vi "Diamond Target Analysis.vi"(10 "gun tracking mode":T1, 11 "Diamond Targets":T4[](array[typedef])) -> (3 "Targetting Output":T3)   [LabVIEW 2011]
uses:
  Diamond Target Output.ctl
  Rectangle Position.ctl
  Target Confidence.ctl
  Camera State.ctl
  gun/gun_tracking_mode.ctl
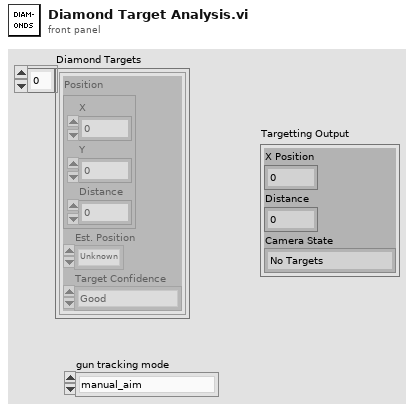
[diagram p1: front panel]
types:
  T1 = typedef "gun_tracking_mode.ctl" = enum16{"manual_aim", "auto_aim_camera", "preset_center_field", "preset_right_pocket", "preset_left_pocket", "align_center", "align_center_backwards", "auto_aim_key", "align_fold", "auton_custom", "preset_pass", "auto_aim_auton"}
  T2 = typedef "Camera State.ctl" = enum16{"No Targets", "Low Confidence", "Medium Confidence", "High Confidence", "Camera Error"}
  T3 = cluster{"X Position":dbl, "Distance":dbl, "Camera State":T2}
  T4 = typedef "Diamond Target Output.ctl" = cluster{"Position":cluster{"X":dbl, "Y":dbl, "Distance":dbl}, "Est. Position":T5, "Target Confidence":T6}
  T5 = typedef "Rectangle Position.ctl" = enum16{"Unknown", "Top", "Right", "Left", "Bottom"}
  T6 = typedef "Target Confidence.ctl" = enum16{"Good", "Good-Clipped Y", "Marginal-Clipped X"}
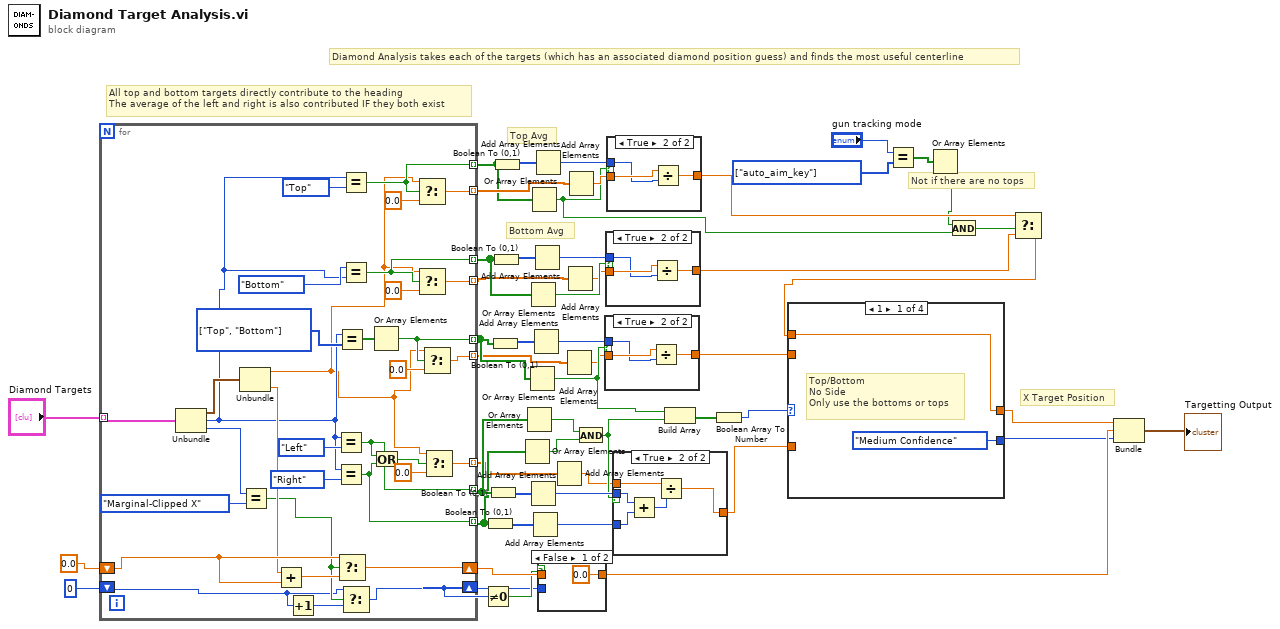
[diagram p0: block diagram]
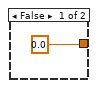
[diagram p2: hidden frame]
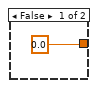
[diagram p3: hidden frame]
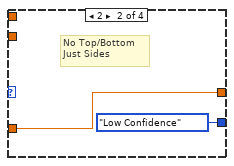
[diagram p4: hidden frame]
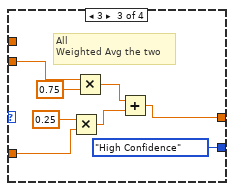
[diagram p5: hidden frame]
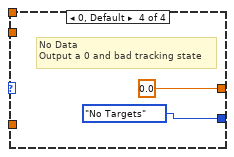
[diagram p6: hidden frame]
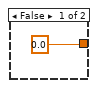
[diagram p7: hidden frame]
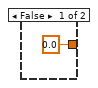
[diagram p8: hidden frame]
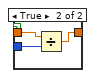
[diagram p9: hidden frame]
diagram:
  w8 = T1[] [enum."auto_aim_key"] items=["manual_aim", "auto_aim_camera", "preset_center_field", "preset_right_pocket", "preset_left_pocket", "align_center", "align_center_backwards", "auto_aim_key", "align_fold", "auton_custom", "preset_pass", "auto_aim_auton"]
  # "Diamond Analysis takes each of the targets (which has an associated diamond position guess) and finds the most useful centerline"
  # "Not if there are no tops"
  # "Top Avg"
  # "Bottom Avg"
  # "X Target Position"
  # "All top and bottom targets directly contribute to the heading\nThe average of the left and right is also contributed IF they both exist"
  n1 = for {
    tunnel: "Diamond Targets" -> [w85] mode=indexing
    tunnel: [w68] -> w37 mode=indexing
    tunnel: [w66] -> w39 mode=indexing
    shift-right: [w77] -> w48
    shift-left: 0.0 -> [w75]
    shift-right: [w73] -> w46
    shift-left: 0 -> [w70]
    tunnel: [w69] -> w38 mode=indexing
    tunnel: [w65] -> w25 mode=indexing
    tunnel: [w63] -> w23 mode=indexing
    tunnel: [w59] -> w15 mode=indexing
    tunnel: [w58] -> w16 mode=indexing
    tunnel: [w54] -> w11 mode=indexing
    tunnel: [w53] -> w10 mode=indexing
    w79 = T5[] [enum."Top", enum."Bottom"] items=["Unknown", "Top", "Right", "Left", "Bottom"]
    n2 = Unbundle(w85) -> ("Position"=w84:cluster{"X":dbl, "Y":dbl, "Distance":dbl}, "Est. Position"=w56:T5, "Target Confidence"=w83:T6)
    n3 = Unbundle(w84) -> ("X"=w52:dbl, "Distance"=w74:dbl)  [unwired: 1 out]
    n4 = Equal?(x=w83, y=Target_Confidence."Marginal-Clipped X") -> (x = y?=w72:bool)
    n5 = Add(x=w74, y=w75) -> (x+y=w76:dbl)
    n6 = Increment(x=w70) -> (x+1=w71:i32)
    n7 = Equal?(x=w56, y=Rectangle_Position."Left") -> (x = y?=w69:bool)
    n8 = Equal?(x=w56, y=Rectangle_Position."Right") -> (x = y?=w68:bool)
    n9 = Equal?(x=w56, y=w79) -> (x = y?=w78:bool[])
    n10 = Select(t=w75, s=w72, f=w76) -> (s? t:f=w77:dbl)
    n11 = Equal?(x=w56, y=Rectangle_Position."Top") -> (x = y?=w53:bool)
    n12 = Equal?(x=Rectangle_Position."Bottom" ("y"), y=w56) -> (x = y?=w58:bool)
    n13 = Select(t=w70, s=w72, f=w71) -> (s? t:f=w73:i32)
    n14 = Or Array Elements(Boolean array=w78) -> (logical OR=w66:bool)
    n15 = Or(x=w69, y=w68) -> (x .or. y?=w67:bool)
    n16 = Select(t=w52, s=w53, f=0.0) -> (s? t:f=w54:dbl)
    n17 = Select(t=w52, s=w58, f=0.0) -> (s? t:f=w59:dbl)
    n18 = Select(t=w52, s=w66, f=0.0) -> (s? t:f=w63:dbl)
    n19 = Select(t=w52, s=w67, f=0.0) -> (s? t:f=w65:dbl)
  }
  n20 = Not Equal To 0?(x=w46) -> (x != 0?=w47:bool)
  n21 = Boolean To (0,1)(Boolean=w37) -> (0, 1=w43:i16[])
  n22 = Boolean To (0,1)(Boolean=w38) -> (0, 1=w44:i16[])
  n23 = Boolean To (0,1)(Boolean=w39) -> (0, 1=w45:i16[])
  n24 = Boolean To (0,1)(Boolean=w16) -> (0, 1=w20:i16[])
  n25 = Boolean To (0,1)(Boolean=w10) -> (0, 1=w14:i16[])
  n26 = Or Array Elements(Boolean array=w37) -> (logical OR=w35:bool)
  n27 = Or Array Elements(Boolean array=w38) -> (logical OR=w36:bool)
  n28 = Or Array Elements(Boolean array=w39) -> (logical OR=w34:bool)
  n29 = Or Array Elements(Boolean array=w16) -> (logical OR=w18:bool)
  n30 = Add Array Elements(numeric array=w44) -> (sum=w41:i16)
  n31 = Or Array Elements(Boolean array=w10) -> (logical OR=w1:bool)
  n32 = Add Array Elements(numeric array=w43) -> (sum=w40:i16)
  n33 = Add Array Elements(numeric array=w45) -> (sum=w42:i16)
  n34 = Add Array Elements(numeric array=w20) -> (sum=w19:i16)
  n35 = Add Array Elements(numeric array=w14) -> (sum=w13:i16)
  n36 = case shown="False" w47 {
    tunnel: w48 -> [_ w89]
    tunnel: w46 -> [_ w88]
    tunnel: [0.0 w87] -> w27
    frame False {
    }
    frame True {
      n37 = Divide(x=w89, y=w88) -> (x/y=w87:dbl)
    }
  }
  n38 = Add Array Elements(numeric array=w25) -> (sum=w24:dbl)
  n39 = Add Array Elements(numeric array=w23) -> (sum=w22:dbl)
  n40 = Add Array Elements(numeric array=w15) -> (sum=w17:dbl)
  n41 = Add Array Elements(numeric array=w11) -> (sum=w12:dbl)
  n42 = And(x=w36, y=w35) -> (x .and. y?=w33:bool)
  n43 = case shown="True" w34 {
    tunnel: w22 -> [_ w93]
    tunnel: w42 -> [_ w92]
    tunnel: [0.0 w91] -> w30
    frame False {
    }
    frame True {
      n44 = Divide(x=w93, y=w92) -> (x/y=w91:dbl)
    }
  }
  n45 = case shown="True" w18 {
    tunnel: w17 -> [_ w97]
    tunnel: w19 -> [_ w96]
    tunnel: [0.0 w95] -> w5
    frame False {
    }
    frame True {
      n46 = Divide(x=w97, y=w96) -> (x/y=w95:dbl)
    }
  }
  n47 = case shown="True" w1 {
    tunnel: w12 -> [_ w101]
    tunnel: w13 -> [_ w100]
    tunnel: [0.0 w99] -> w6
    frame False {
    }
    frame True {
      n48 = Divide(x=w101, y=w100) -> (x/y=w99:dbl)
    }
  }
  n49 = case shown="True" w33 {
    tunnel: w41 -> [_ w107]
    tunnel: w40 -> [_ w106]
    tunnel: [0.0 w103] -> w29
    tunnel: w24 -> [_ w104]
    frame False {
    }
    frame True {
      n50 = Add(x=w107, y=w106) -> (x+y=w105:i16)
      n51 = Divide(x=w104, y=w105) -> (x/y=w103:dbl)
    }
  }
  n52 = Build Array(w34, w33) -> (w32:bool[])
  n53 = Boolean Array To Number(Boolean array=w32) -> (number=w31:u32)
  n54 = Equal?(x="gun tracking mode", y=w8) -> (x = y?=w7:bool[])
  n55 = Or Array Elements(Boolean array=w7) -> (logical OR=w2:bool)
  n56 = And(x=w2, y=w1) -> (x .and. y?=w3:bool)
  n57 = Select(t=w6, s=w3, f=w5) -> (s? t:f=w4:dbl)
  n58 = case shown="1" w31 {
    tunnel: [Camera_State."Medium Confidence" ("Camera State") Camera_State."Low Confidence" ("Camera State") Camera_State."High Confidence" ("Camera State") Camera_State."No Targets" ("Camera State")] -> w26
    tunnel: [w108 w110 w112 0.0] -> w28
    tunnel: w30 -> [_ _ w118 _]
    tunnel: w29 -> [_ w110 w115 _]
    tunnel: w4 -> [w108 _ _ _]
    frame 1 {
      # "Top/Bottom\nNo Side\nOnly use the bottoms or tops"
    }
    frame 2 {
      # "No Top/Bottom\nJust Sides"
    }
    frame 3 {
      # "All\nWeighted Avg the two"
      n59 = Multiply(x=0.25, y=w115) -> (x*y=w113:dbl)
      n60 = Multiply(x=w118, y=0.75) -> (x*y=w114:dbl)
      n61 = Add(x=w114, y=w113) -> (x+y=w112:dbl)
    }
    frame 0, Default {
      # "No Data\nOutput a 0 and bad tracking state"
    }
  }
  n62 = Bundle(w28, w27, "Camera State"=w26) -> (→"Targetting Output":cluster{dbl, dbl, "Camera State":T2})  [unwired: 1 in]
